vi "EOL CAN_Stop CAN.vi"(8 "error in (no error)":errorcluster, 11 "XNET Session Array In":refnum<k21>[](array[refnum])) -> (0 "error out":errorcluster)   [LabVIEW 2014]
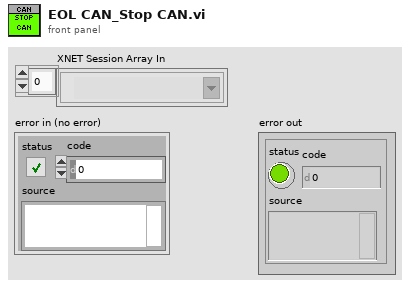
[diagram p1: front panel]
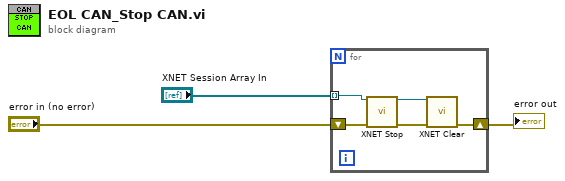
[diagram p0: block diagram]
diagram:
  n1 = for {
    shift-right: [w5] -> w2
    shift-left: "error in (no error)" -> [w6]
    tunnel: "XNET Session Array In" -> [w4] mode=indexing
    n2 = call <vilib>:"XNET Stop.vi"("session in"=w4, "error in (no error)"=w6) -> ("session out"=w7:refnum<k21>, "error out"=w8:errorcluster)  [unwired: 12 in]
    n3 = call <vilib>:"XNET Clear.vi"("session in"=w7, "error in (no error)"=w8) -> ("error out"=w5:errorcluster)  [unwired: 13 in]
  }
  "error out" <- w2
